vi "set_trigger_delay.vi"() -> ()   [LabVIEW 2020]
panel:
  out "display file":string
  in  "Path":path
  out "display m3510A":string
  in  "Voltmeter Picotest M3510A":refnum<visa-resource-name>
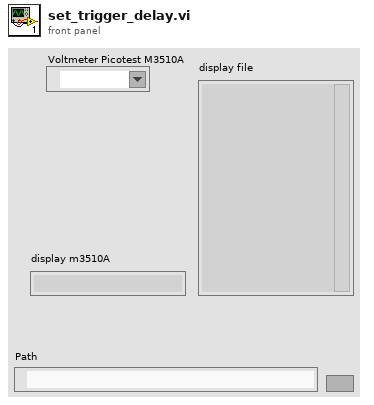
[diagram p1: front panel]
types:
  T1 = enum16{"read/write", "read-only", "write-only", ""}
  T2 = enum16{"open", "replace", "create", "open or create", "replace or create", "replace or create with confirmation", ""}
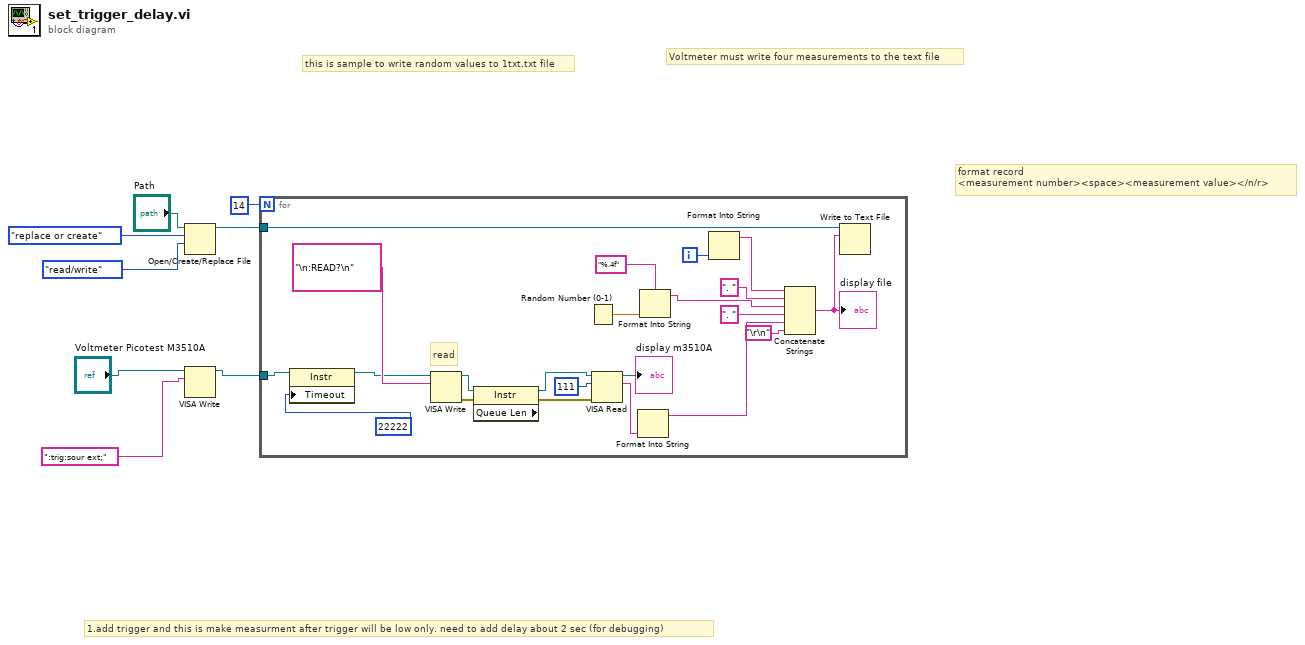
[diagram p0: block diagram]
diagram:
  # "1.add trigger and this is make measurment after trigger will be low only. need to add delay about 2 sec (for debugging)"
  # "format record \n<measurement number><space><measurement value></n/r>"
  # "Voltmeter must write four measurements to the text file"
  # "this is sample to write random values to 1txt.txt file"
  n1 = Open/Create/Replace File(file path (use dialog)="Path", operation (0:open)=T2."replace or create", access (0:read/write)=T1."read/write") -> (refnum out=w4:refnum<file>)  [unwired: 3 in, 2 out]
  n2 = VISA Write(VISA resource name="Voltmeter Picotest M3510A", write buffer=":trig:sour ext;") -> (VISA resource name out=w3:refnum<visa-resource-name>)  [unwired: 1 in, 2 out]
  n3 = for {
    N: 14 -> [_]
    tunnel: w3 -> [w11]
    tunnel: w4 -> [w13]
    i -> [w24]
    # "read"
    n4 = property class="Instr"(reference=w11, "Timeout"=22222) -> (reference out=w10:refnum<visa-resource-name>)  [unwired: 1 in, 1 out]
    n5 = VISA Write(VISA resource name=w10, write buffer="\n:READ?\n") -> (VISA resource name out=w28:refnum<visa-resource-name>, error out=w29:errorcluster)  [unwired: 1 in, 1 out]
    n6 = property class="Instr" props=["Queue Len"](reference=w28, error in=w29) -> (reference out=w27:refnum<visa-resource-name>, error out=w26:errorcluster)  [unwired: 1 out]
    n7 = Random Number (0-1)() -> (number: 0 to 1=w25:dbl)
    n8 = VISA Read(VISA resource name=w27, byte count=111, error in (no error)=w26) -> (VISA resource name out=→"display m3510A":refnum<visa-resource-name>, read buffer=w15:string)  [unwired: 2 out]
    n9 = Format Into String(w15) -> (resulting string=w17:string)  [unwired: 3 in, 1 out]
    n10 = Format Into String(format string="%.4f", w25) -> (resulting string=w21:string)  [unwired: 2 in, 1 out]
    n11 = Format Into String(w24) -> (resulting string=w23:string)  [unwired: 3 in, 1 out]
    n12 = Concatenate Strings(w23, ". ", w21, ". ", w17, "\r\n") -> (w14:string)
    "display file" <- w14
    n13 = Write to Text File(file (use dialog)=w13, text=w14) -> ()  [unwired: 2 in, 3 out]
  }
